vi "Global Strings.vi"() -> ()   [LabVIEW 2011, in "BK Precision 91xx (GPIB) Custom Device.lvlib"]
uses:
  BK Precision 91xx (GPIB) Custom Device.lvlib
panel:
  in  "Serial":string="Serial"
  in  "FilterTimeoutError":string="FilterTimeoutError"
  in  "ID Query":string="ID Query"
  in  "Update Rate":string="Update Rate"
  in  "Visa Resource Name":string="Visa Resource Name"
  in  "Voltage Limit":string="Voltage Limit"
  in  "Enable OVP":string="Enable OVP"
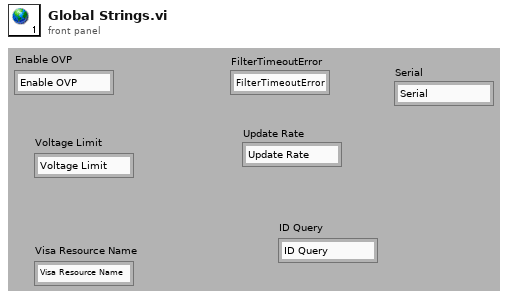
[diagram p1: front panel]
diagram:
